vi "close.vi"(8 "error in":errorcluster, 11 "bin datalogger runtime in":refnum<class "Binary datalogger runtime.lvclass">) -> (0 "error out":errorcluster)   [LabVIEW 2013, in "Binary datalogger runtime.lvclass"]
doc: "Provides an interface for terminating a module instance. While this interface performs no operations, a child should close and deallocate any open references or memory."
uses:
  Binary datalogger runtime.lvclass
  Binary datalogger runtime.lvclass/Binary datalogger runtime.ctl
  message to background process.ctl
  control enum.ctl
  <vilib>/NI/Tag Bus/table/data table.ctl
  <vilib>/NI/Tag Bus/table/data table.lvlib
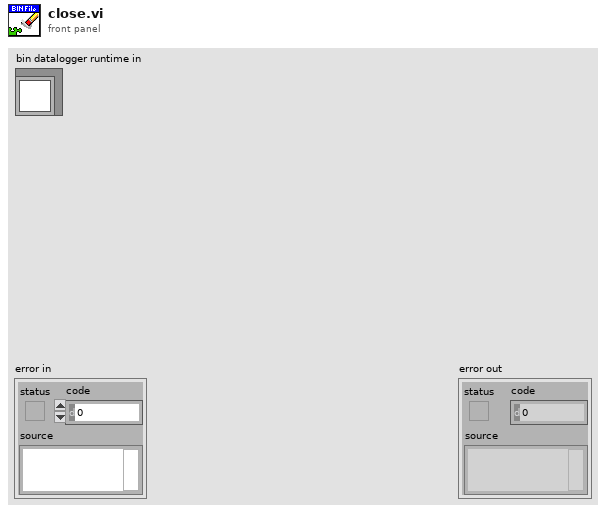
[diagram p1: front panel]
types:
  T1 = typedef "Binary datalogger runtime.lvclass/control enum.ctl" = enum16{"exit", "output data"}
  T2 = typedef "Binary datalogger runtime.lvclass/message to background process.ctl" = cluster{"control enum":T1, "datapack":refnum<data-value>, "Time Stamp":timestamp}
  T3 = typedef "TDMS datalogger runtime.lvclass/response from background process.ctl" = cluster{"response enum":T4, "datapack":refnum<data-value>, "error code":i32}
  T4 = typedef "TDMS datalogger runtime.lvclass/response enum.ctl" = enum16{"exit", "return buffer", "error"}
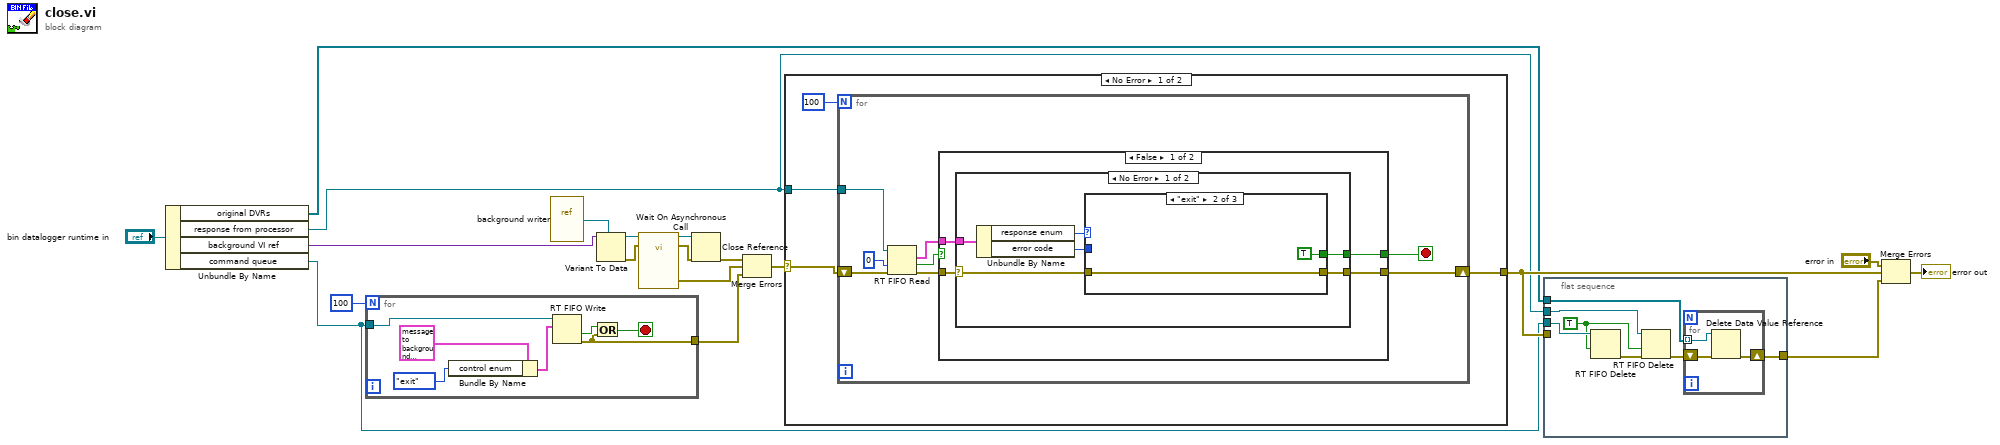
[diagram p0: block diagram]
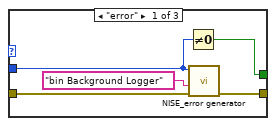
[diagram p2: hidden frame]
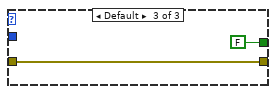
[diagram p3: hidden frame]
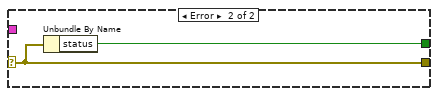
[diagram p4: hidden frame]
diagram:
  n1 = Unbundle By Name("bin datalogger runtime in") -> ("original DVRs"=w2:refnum<data-value>[], "response from processor"=w3:refnum<k33>, "background VI ref"=w15:variant, "command queue"=w4:refnum<k33>)
  n2 = for {
    N: 100 -> [_]
    tunnel: w4 -> [w26]
    tunnel: [w20] -> w7
    stop <- w21 stop-if-true
    n3 = Bundle By Name(cluster=T2 {"control enum"=enum."exit", "datapack"=refnum, "Time Stamp"=timestamp(0 s since 1904-01-01)} ("element"), "control enum"=control_enum."exit") -> (w24:T2)
    n4 = RT FIFO Write(0:w26, 1:w24) -> (10:w22:bool, 11:w20:errorcluster)  [unwired: 3 in, 2 out]
    n5 = Or(x=w22, y=w20) -> (x .or. y?=w21:bool)
  }
  n6 = vi-ref "background writer.vi"() -> (w16:refnum<vi>)
  n7 = Variant To Data(type=w16, Variant=w15) -> (data=w12:refnum<vi>, error out=w13:errorcluster)  [unwired: 1 in]
  n8 = call-by-ref "Wait On Asynchronous Call"(reference=w12, error in=w13) -> (reference out=w10:refnum<vi>, error out=w11:errorcluster, 15:"error out"=w8:errorcluster)  [unwired: 15 in]
  n9 = Close Reference(reference=w10, error in (no error)=w11) -> (error out=w9:errorcluster)
  n10 = Merge Errors(w9, w8, w7) -> (w6:errorcluster)
  n11 = case shown="No Error" w6 {
    selector: w6 -> [w28 w62]
    tunnel: [w27 w62] -> w5
    tunnel: w3 -> [w29 _]
    frame No Error {
      n12 = for {
        N: 100 -> [_]
        tunnel: w29 -> [w38]
        shift-right: [w34] -> w27
        shift-left: w28 -> [w37]
        stop <- w32 stop-if-true
        n13 = RT FIFO Read(0:w38, 2:0 ("timeout in ms (0)"), 3:w37) -> (9:w31:T3, 10:w35:bool, 11:w33:errorcluster)  [unwired: 1 in, 2 out]
        n14 = case shown="False" w35 {
          selector: w35 -> [_ w60]
          tunnel: [w41 w61] -> w34
          tunnel: w33 -> [w42 w61]
          tunnel: [w40 w60] -> w32
          tunnel: w31 -> [w39 _]
          frame False {
            n15 = case shown="No Error" w42 {
              selector: w42 -> [w45 w59]
              tunnel: [w46 w59] -> w41
              tunnel: [w44 w58] -> w40
              tunnel: w39 -> [w48 _]
              frame No Error {
                n16 = Unbundle By Name(w48) -> ("response enum"=w47:T4, "error code"=w43:i32)
                n17 = case shown="\"exit\"" w47 {
                  tunnel: [w52 w55 w57] -> w46
                  tunnel: w45 -> [w53 w55 w57]
                  tunnel: [w50 TRUE FALSE] -> w44
                  tunnel: w43 -> [w49 _ _]
                  frame "error" {
                    n18 = Not Equal To 0?(x=w49) -> (x != 0?=w50:bool)
                    n19 = call <vilib>:"NISE_error generator.vi"("error in"=w53, "source"="bin Background Logger", "error code (0)"=w49) -> ("error out"=w52:errorcluster)  [unwired: 6 in]
                  }
                  frame "exit" {
                  }
                  frame Default {
                  }
                }
              }
              frame Error {
                n20 = Unbundle By Name(w59) -> ("status"=w58:bool)
              }
            }
          }
          frame True {
          }
        }
      }
    }
    frame Error {
      # "don't need even more errors"
    }
  }
  n21 = flat-sequence {
    tunnel: w5 -> [_]
    tunnel: w4 -> [w69]
    tunnel: w3 -> [w68]
    tunnel: w2 -> [w64]
    tunnel: [w63] -> w1
    frame #0 {
      w66 = TRUE ("force destroy? (F)")
      n22 = RT FIFO Delete(0:w69, 2:w66) -> (11:w67:errorcluster)  [unwired: 1 in]
      n23 = RT FIFO Delete(0:w68, 2:w66, 3:w67) -> (11:w65:errorcluster)
      n24 = for {
        tunnel: w64 -> [w71] mode=indexing
        shift-right: [w70] -> w63
        shift-left: w65 -> [w72]
        n25 = Delete Data Value Reference(data value reference=w71, error in=w72) -> (error out=w70:errorcluster)  [unwired: 1 out]
      }
    }
  }
  n26 = Merge Errors("error in", w5, w1) -> (→"error out":errorcluster)
